vi "RecordDataReader.vi"(6 "format":i32=212, 8 "error in":errorcluster, 9 "No of signals(1)":i32=1, 11 "File refnum in":refnum<file>) -> (0 "error out":errorcluster, 2 "Signals":i16[][](array[numeric]), 3 "File refnum out":refnum<file>)   [LabVIEW 2012]
doc: "Reads information from data file, being a part of Physionet record. <b>File refnum in</b> must be a reference to an already opened file. <b>File refnum out</b> is its duplicate. <b>No of signals(1)</b> indicates how many signals are contained in the file. <b>Signals</b> is a N-row array, where N is number of signals read. Its number of columns equals signals' lengths."
panel:
  in  "file (use dialog)":path
  out "SamplesPerSignal":i32
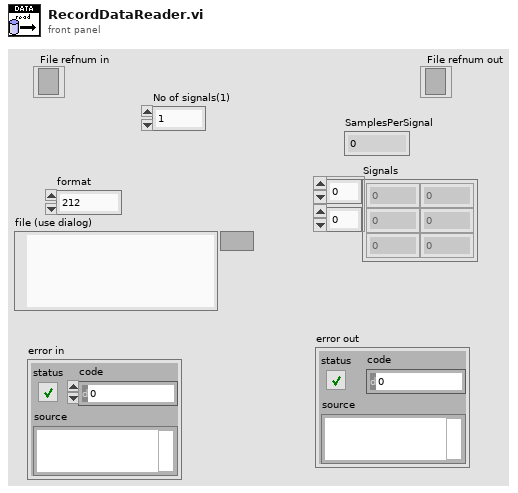
[diagram p1: front panel]
types:
  T1 = enum16{"big-endian, network order", "native, host order", "little-endian"}
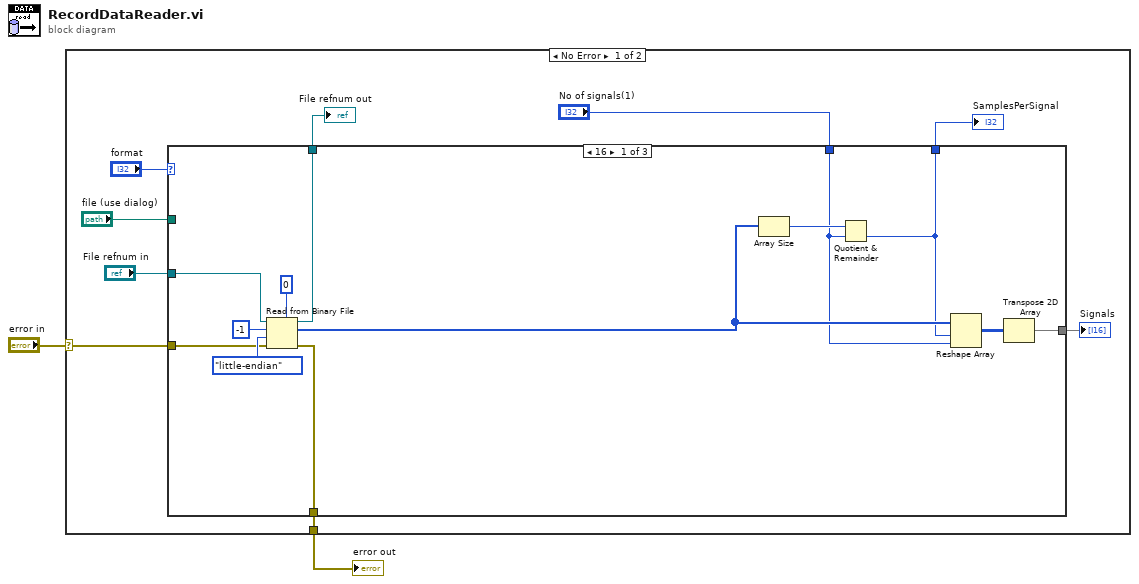
[diagram p0: block diagram]
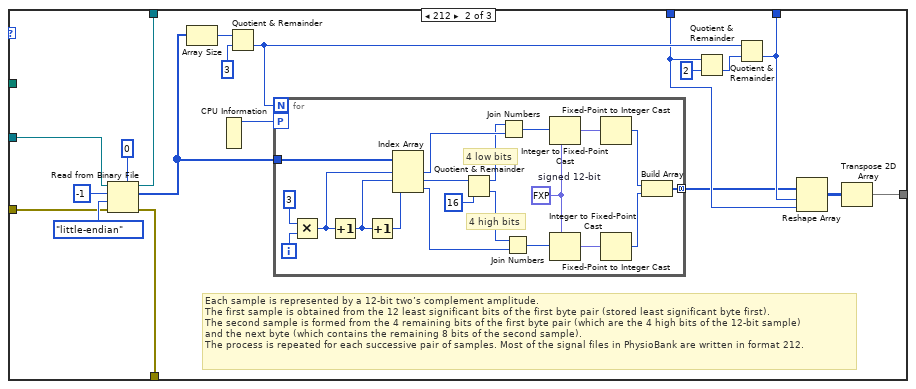
[diagram p2: hidden frame]
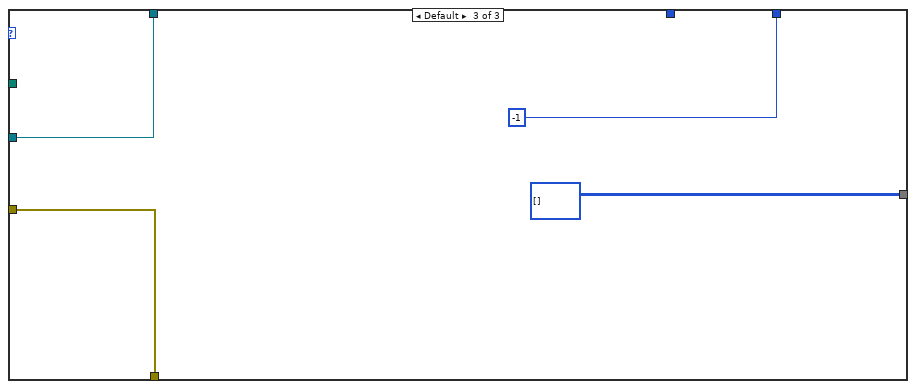
[diagram p3: hidden frame]
diagram:
  n1 = case shown="No Error" "error in" {
    selector: "error in" -> [w10 w68]
    tunnel: [w5 w68] -> w2
    frame No Error {
      n2 = case shown="16" "format" {
        tunnel: [w14 w32 -1] -> w11
        tunnel: [w12 w25 i16[][] []] -> w3
        tunnel: w10 -> [w23 w37 w65]
        tunnel: [w21 w36 w64] -> w8
        tunnel: "file (use dialog)" -> [_ _ _]
        tunnel: "File refnum in" -> [w16 w30 w64]
        tunnel: [w20 w31 w65] -> w5
        tunnel: "No of signals(1)" -> [w13 w27 _]
        frame 16 {
          n3 = Read from Binary File(5:i16 0, 8:w23, 9:T1."little-endian" ("byte order (0:big-endian, network order)"), 10:-1 ("count (1)"), 11:w16) -> (0:w20:errorcluster, 2:w18:i16[], 3:w21:refnum<file>)  [unwired: 1 in, 1 out]
          n4 = Array Size(array=w18) -> (size(s)=w15:i32)
          n5 = Quotient & Remainder(x=w15, y=w13) -> (floor(x/y)=w14:i32)  [unwired: 1 out]
          n6 = Reshape Array(w18, w14, w13) -> (w19:i16[][])
          n7 = Transpose 2D Array(2D array=w19) -> (transposed array=w12:i16[][])
        }
        frame 212 {
          # "Each sample is represented by a 12-bit two’s complement amplitude. \nThe first sample is obtained from the 12 least significant bits of the first byte pair (stored least significant byte first). \nThe second sample is formed from the 4 remaining bits of the first byte pair (which are the 4 high bits of the 12-bit sample) \nand the next byte (which contains the remaining 8 bits of the second sample). \nThe process is repeated for each successive pair of samples. Most of the signal files in PhysioBank are written in format 212."
          n8 = Read from Binary File(5:u8 0, 8:w37, 9:T1."little-endian" ("byte order (0:big-endian, network order)"), 10:-1 ("count (1)"), 11:w30) -> (0:w31:errorcluster, 2:w38:u8[], 3:w36:refnum<file>)  [unwired: 1 in, 1 out]
          n9 = Array Size(array=w38) -> (size(s)=w43:i32)
          n10 = CPU Information() -> (4:w41:i32)  [unwired: 3 out]
          n11 = Quotient & Remainder(x=w43, y=3) -> (floor(x/y)=w33:i32)  [unwired: 1 out]
          n12 = for {
            N: w33 -> [_]
            tunnel: w38 -> [w58]
            workers-P: w41 -> [_]
            tunnel: [w44] -> w26 mode=concatenating
            i -> [w63]
            w47 = fxp<+/-,12,12> 0.0  # signed 12-bit
            # "4 low bits"
            # "4 high bits"
            n13 = Multiply(x=3 ("y"), y=w63) -> (x*y=w61:i32)
            n14 = Increment(x=w61) -> (x+1=w60:i32)
            n15 = Increment(x=w60) -> (x+1=w59:i32)
            n16 = Index Array(array=w58, index #1=w61, index #2=w60, index #3=w59) -> (element #1=w56:u8, element #2=w55:u8, element #3=w54:u8)
            n17 = Quotient & Remainder(x=w55, y=u8 16) -> (x-y*floor(x/y)=w50:u8, floor(x/y)=w49:u8)
            n18 = Join Numbers(hi=w50, lo=w56) -> ((hi.lo)=w57:u16)
            n19 = Join Numbers(hi=w49, lo=w54) -> ((hi.lo)=w51:u16)
            n20 = Integer to Fixed-Point Cast(fixed-point type=w47, integer=w57) -> (fixed-point=w53:fxp<+/-,12,12>)
            n21 = Integer to Fixed-Point Cast(fixed-point type=w47, integer=w51) -> (fixed-point=w52:fxp<+/-,12,12>)
            n22 = Fixed-Point to Integer Cast(1:w53) -> (0:w46:i16)
            n23 = Fixed-Point to Integer Cast(1:w52) -> (0:w45:i16)
            n24 = Build Array(w46, w45) -> (w44:i16[])
          }
          n25 = Quotient & Remainder(x=w27, y=2) -> (floor(x/y)=w29:i32)  [unwired: 1 out]
          n26 = Quotient & Remainder(x=w33, y=w29) -> (floor(x/y)=w32:i32)  [unwired: 1 out]
          n27 = Reshape Array(w26, w32, w27) -> (w28:i16[][])
          n28 = Transpose 2D Array(2D array=w28) -> (transposed array=w25:i16[][])
        }
        frame Default {
        }
      }
      "SamplesPerSignal" <- w11
      "Signals" <- w3
      "File refnum out" <- w8
    }
    frame Error {
    }
  }
  "error out" <- w2
